vi "valid form.vi"(11 "User Information":T1 {"Country" items=["Afghanistan", "Aland Islands", "Albania", "Algeria", "American Samoa", "Andorra", "Angola", "Anguilla", "Antarctica", "Antigua And Barbuda", "Argentina", "Armenia", "Aruba", "Australia", "Austria", "Azerbaijan", "Bahamas", "Bahrain", "Bangladesh", "Barbados", "Belarus", "Belgium", "Belize", "Benin", "Bermuda", "Bhutan", "Bolivia", "Bosnia And Herzegovina", "Botswana", "Bouvet Island", "Brazil", "British Indian Ocean Territory", "Brunei Darussalam", "Bulgaria", "Burkina Faso", "Burundi", "Cambodia", "Cameroon", "Canada", "Cape Verde", "Cayman Islands", "Central African Republic", "Chad", "Chile", "China", "Christmas Island", "Cocos (Keeling) Islands", "Colombia", "Comoros", "Congo", "Congo, The Democratic Republic Of The", "Cook Islands", "Costa Rica", "Cote D'Ivoire", "Croatia", "Cuba", "Cyprus", "Czech Republic", "Denmark", "Djibouti", "Dominica", "Dominican Republic", "Ecuador", "Egypt", "El Salvador", "Equatorial Guinea", "Eritrea", "Estonia", "Ethiopia", "Falkland Islands (Malvinas)", "Faroe Islands", "Fiji", "Finland", "France", "French Guiana", "French Polynesia", "French Southern Territories", "Gabon", "Gambia", "Georgia", "Germany", "Ghana", "Gibraltar", "Greece", "Greenland", "Grenada", "Guadeloupe", "Guam", "Guatemala", "Guernsey", "Guinea", "Guinea-Bissau", "Guyana", "Haiti", "Heard Island And Mcdonald Islands", "Holy See (Vatican City State)", "Honduras", "Hong Kong", "Hungary", "Iceland", "India", "Indonesia", "Iran, Islamic Republic Of", "Iraq", "Ireland", "Isle Of Man", "Israel", "Italy", "Jamaica", "Japan", "Jersey", "Jordan", "Kazakhstan", "Kenya", "Kiribati", "Korea, Democratic People'S Republic Of", "Korea, Republic Of", "Kuwait", "Kyrgyzstan", "Lao People'S Democratic Republic", "Latvia", "Lebanon", "Lesotho", "Liberia", "Libyan Arab Jamahiriya", "Liechtenstein", "Lithuania", "Luxembourg", "Macao", "Macedonia, The Former Yugoslav Republic Of", "Madagascar", "Malawi", "Malaysia", "Maldives", "Mali", "Malta", "Marshall Islands", "Martinique", "Mauritania", "Mauritius", "Mayotte", "Mexico", "Micronesia, Federated States Of", "Moldova, Republic Of", "Monaco", "Mongolia", "Montserrat", "Morocco", "Mozambique", "Myanmar", "Namibia", "Nauru", "Nepal", "Netherlands", "Netherlands Antilles", "New Caledonia", "New Zealand", "Nicaragua", "Niger", "Nigeria", "Niue", "Norfolk Island", "Northern Mariana Islands", "Norway", "Oman", "Pakistan", "Palau", "Palestinian Territory, Occupied", "Panama", "Papua New Guinea", "Paraguay", "Peru", "Philippines", "Pitcairn", "Poland", "Portugal", "Puerto Rico", "Qatar", "Reunion", "Romania", "Russian Federation", "Rwanda", "Saint Helena", "Saint Kitts And Nevis", "Saint Lucia", "Saint Pierre And Miquelon", "Saint Vincent And The Grenadines", "Samoa", "San Marino", "Sao Tome And Principe", "Saudi Arabia", "Senegal", "Serbia And Montenegro", "Seychelles", "Sierra Leone", "Singapore", "Slovakia", "Slovenia", "Solomon Islands", "Somalia", "South Africa", "South Georgia And The South Sandwich Islands", "Spain", "Sri Lanka", "Sudan", "Suriname", "Svalbard And Jan Mayen", "Swaziland", "Sweden", "Switzerland", "Syrian Arab Republic", "Taiwan, Province Of China", "Tajikistan", "Tanzania, United Republic Of", "Thailand", "Timor-Leste", "Togo", "Tokelau", "Tonga", "Trinidad And Tobago", "Tunisia", "Turkey", "Turkmenistan", "Turks And Caicos Islands", "Tuvalu", "Uganda", "Ukraine", "United Arab Emirates", "United Kingdom", "United States", "United States Minor Outlying Islands", "Uruguay", "Uzbekistan", "Vanuatu", "Venezuela", "Viet Nam", "Virgin Islands, British", "Virgin Islands, U.S.", "Wallis And Futuna", "Western Sahara", "Yemen", "Zambia", "Zimbabwe", "(Not Specified)"]}) -> (3 "valid form":bool)   [LabVIEW 2015, in "AguaClara Library.lvlib"]
uses:
  AguaClara Library.lvlib
  User Information.ctl
  Country Ring.ctl
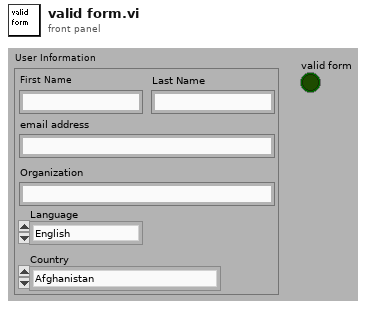
[diagram p1: front panel]
types:
  T1 = typedef "AguaClara Library.lvlib/User Information.ctl" = cluster{"First Name":string, "Last Name":string, "Email Address":string, "Organization":string, "Language":enum16{"English", "Español", "French"}, "Country":T2}
  T2 = typedef "Country Ring.ctl" = u16
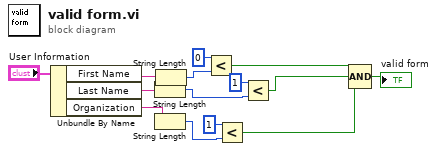
[diagram p0: block diagram]
diagram:
  n1 = Unbundle By Name("User Information") -> ("First Name"=w13:string, "Last Name"=w12:string, "Organization"=w11:string)
  n2 = String Length(string=w12) -> (length=w7:i32)
  n3 = String Length(string=w11) -> (length=w5:i32)
  n4 = String Length(string=w13) -> (length=w10:i32)
  n5 = Less?(x=0, y=w10) -> (x < y?=w4:bool)
  n6 = Less?(x=1, y=w5) -> (x < y?=w2:bool)
  n7 = Less?(x=1, y=w7) -> (x < y?=w3:bool)
  n8 = Compound Arithmetic op=AND(w4, w3, w2) -> (→"valid form":bool)
